vi "KE622x -- Arm Init Delta Meas.vi"(0 "Resource In":refnum<visa-resource-name>, 1 "Check For SCPI Errors? (T)":bool=TRUE, 11 "error in (no error)":errorcluster) -> (4 "Resource Out (dupl)":refnum<visa-resource-name>, 15 "error out":errorcluster)   [LabVIEW 2010, in "Keithley 622x.lvlib"]
uses:
  Keithley 622x.lvlib
panel:
  in  "Init Delta Meas? (T)":bool=TRUE
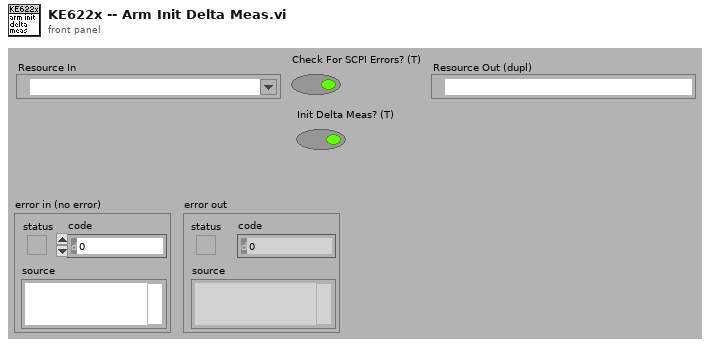
[diagram p1: front panel]
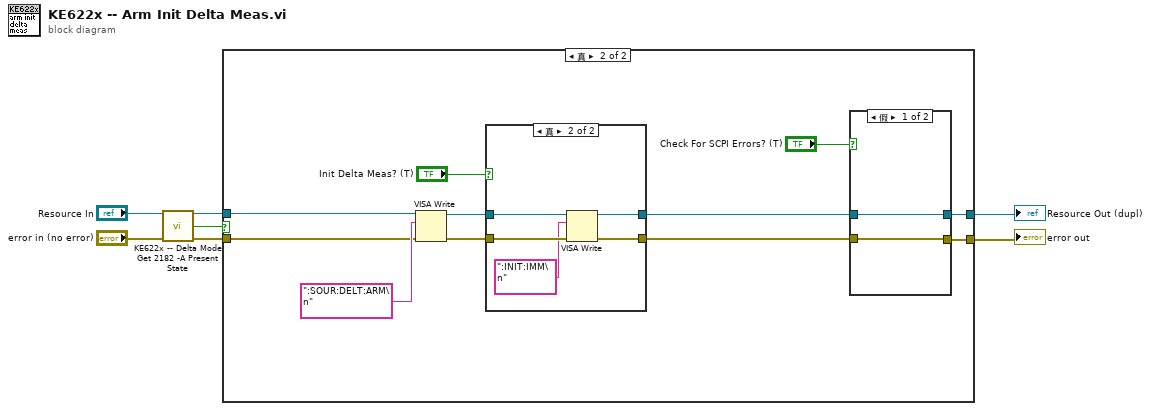
[diagram p0: block diagram]
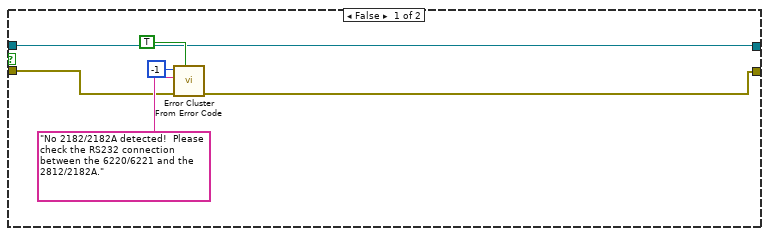
[diagram p2: hidden frame]
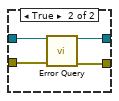
[diagram p4: hidden frame]
diagram:
  n1 = call "KE622x -- Delta Mode Get 2182 -A Present State.vi"("Resource In"="Resource In", "error in (no error)"="error in (no error)") -> ("Resource Out (dupl)"=w3:refnum<visa-resource-name>, "2182/2182A Present?"=w5:bool, "error out"=w4:errorcluster)  [unwired: 11 in]
  n2 = case shown="真" w5 {
    tunnel: w4 -> [w11 w22]
    tunnel: w3 -> [w8 w21]
    tunnel: [w8 w15] -> w2
    tunnel: [w9 w14] -> w1
    frame False {
      n3 = call <vilib>:"Error Cluster From Error Code.vi"("show call chain? (False)"=TRUE, "error in (no error)"=w11, "error message (\"\")"="No 2182/2182A detected!  Please check the RS232 connection between the 6220/6221 and the 2812/2182A.", "error code (0)"=-1) -> ("error out"=w9:errorcluster)  [unwired: 5 in]
    }
    frame True {
      n4 = VISA Write(VISA resource name=w21, write buffer=":SOUR:DELT:ARM\n" ("format string"), error in (no error)=w22) -> (VISA resource name out=w19:refnum<visa-resource-name>, error out=w18:errorcluster)  [unwired: 1 out]
      n5 = case shown="真" "Init Delta Meas? (T)" {
        tunnel: w19 -> [w26 w31]
        tunnel: w18 -> [w25 w30]
        tunnel: [w25 w28] -> w17
        tunnel: [w26 w27] -> w16
        frame False {
        }
        frame True {
          n6 = VISA Write(VISA resource name=w31, write buffer=":INIT:IMM\n", error in (no error)=w30) -> (VISA resource name out=w27:refnum<visa-resource-name>, error out=w28:errorcluster)  [unwired: 1 out]
        }
      }
      n7 = case shown="假" "Check For SCPI Errors? (T)" {
        tunnel: w16 -> [w33 w37]
        tunnel: w17 -> [w32 w36]
        tunnel: [w32 w35] -> w14
        tunnel: [w33 w34] -> w15
        frame False {
        }
        frame True {
          n8 = call "Error Query.vi"("VISA Resource In"=w37, "error in (no error)"=w36) -> ("VISA Resource Out (dupl)"=w34:refnum<visa-resource-name>, "error out"=w35:errorcluster)  [unwired: 10 in, 2 out]
        }
      }
    }
  }
  "Resource Out (dupl)" <- w2
  "error out" <- w1
